vi "ATMEGA_Read_Write_labview.vi"() -> ()   [LabVIEW 2013]
doc: "This example performs writes and reads on a serial port, as directed by the user. You can press the Write and Read buttons, and change the Read Count, while the example is running.\n\nThe parameters set for the serial port must match the parameters of the connected instrument or device. In this example, the Read Count parameter specifies the number of bytes that the serial port reads. If there were more bytes at the port than the specified number, those bytes would not be read. If there were less bytes at the port than the specified number, you would receive a timeout error.\n\nThis example expands upon the flow control options for XON and XOFF, allowing the user to choose those control characters. Also, the user can enable or disable a termination character. Some devices require a termination character in order to identify the end of command strings. Some devices send a termination character to signify the end of data to be read. This example shows how you can end the Read operation once a termination character is detected in the buffer and/or append a termination character at the end of the Write data."
uses:
  D:/Program Files (x86)/National Instruments/LabVIEW 2013/examples/Instrument IO/Serial/support/Serial - Settings.ctl
  <vilib>/Instr/_visa.llb/VISA Configure Serial Port (Instr).vi
panel:
  out "Thermometer":dbl(slide) scale=0.0..500.0
  out "TEMP":i32
  out "READ BUFFER":string
  in  "write buffer":string
  in  "Stop":bool
  in  "Read Count":u32=1000
  out "Response":string
  in  "Write":bool
  in  "Read":bool
  in  "Serial Settings":T1={"baud rate"=9600, "data bits"=8, "parity"=enum."None", "stop bits"=10, "flow control"=0} {"flow control" items=["None"=0, "XON/XOFF"=1, "RTS/CTS"=2, "DTR/DSR"=4]; "stop bits" items=["1.0"=10, "1.5"=15, "2.0"=20]; "data bits" min=5 max=8 step=1; "baud rate" items=["75"=75, "110"=110, "134"=134, "150"=150, "300"=300, "600"=600, "1200"=1200, "1800"=1800, "2400"=2400, "4800"=4800, "7200"=7200, "9600"=9600, "14400"=14400, "19200"=19200, "28800"=28800, "38400"=38400, "56000"=56000, "57600"=57600, "115200"=115200, "128000"=128000, "230400"=230400]}
  in  "VISA resource name":refnum<visa-resource-name>="COM1"
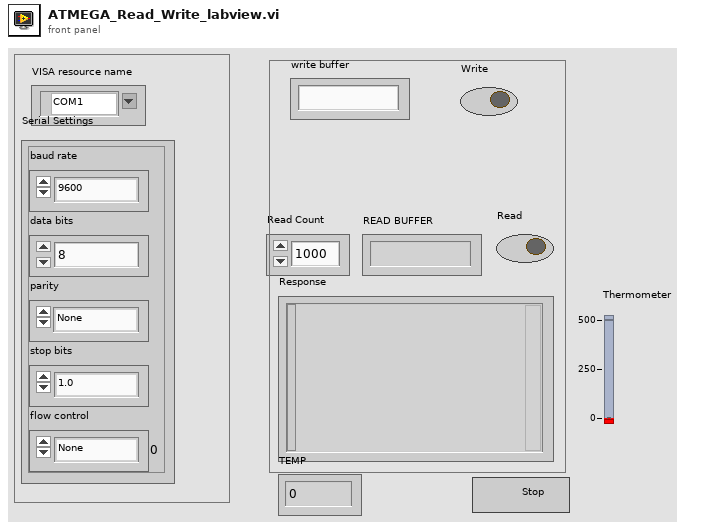
[diagram p1: front panel]
types:
  T1 = typedef "Serial - Settings.ctl" = cluster{"baud rate":u32, "data bits":u16, "parity":enum16{"None", "Odd", "Even", "Mark", "Space"}, "stop bits":u16, "flow control":u16}
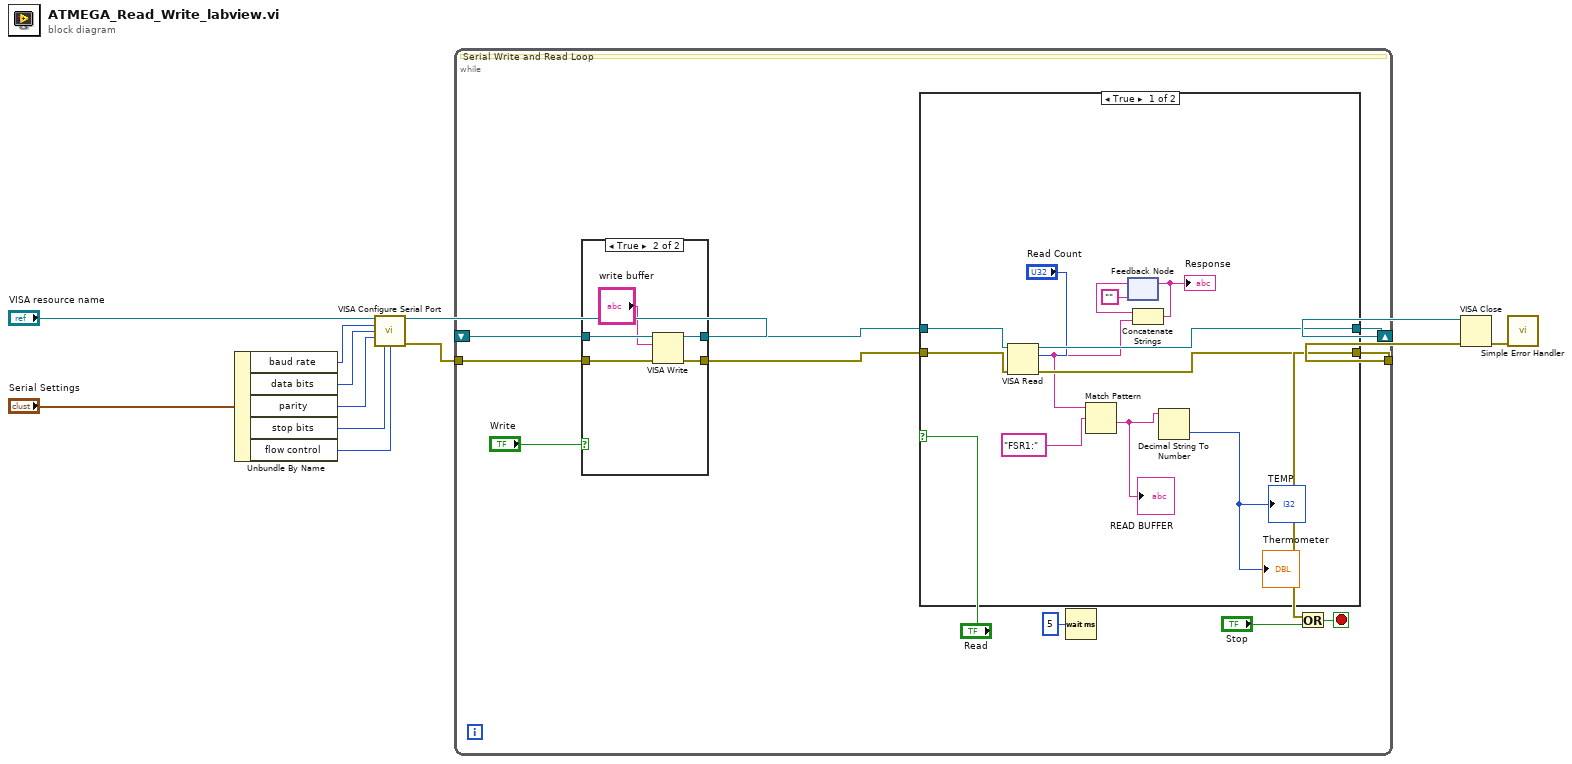
[diagram p0: block diagram]
diagram:
  n1 = Unbundle By Name "Unbundle By Name"("Serial Settings") -> ("baud rate"=w8:u32, "data bits"=w9:u16, "parity"=w10:enum16{"None", "Odd", "Even", "Mark", "Space"}, "stop bits"=w11:u16, "flow control"=w3:u16)
  n2 = call-poly "VISA Configure Serial Port"("VISA resource name"="VISA resource name", "baud rate (9600)"=w8, "data bits (8)"=w9, "parity (0:none)"=w10, "stop bits (10: 1 bit)"=w11, "flow control (0:none)"=w3) -> ("VISA resource name out"=w2:refnum<visa-resource-name>, "error out"=w1:errorcluster)  [unwired: 4 in, 4 out]
  n3 = while {
    shift-right: [w23] -> w4
    shift-left: w2 -> [w22]
    tunnel: [w16] -> w5
    tunnel: w1 -> [w13]
    stop <- w17 stop-if-true
    # "Serial Write and Read Loop"
    n4 = case shown="True" "Write" {
      tunnel: w22 -> [w25 w30]
      tunnel: w13 -> [w24 w29]
      tunnel: [w25 w28] -> w21
      tunnel: [w24 w27] -> w20
      frame False {
      }
      frame True {
        n5 = VISA Write(VISA resource name=w30, write buffer="write buffer", error in (no error)=w29) -> (VISA resource name out=w28:refnum<visa-resource-name>, error out=w27:errorcluster)  [unwired: 1 out]
      }
    }
    n6 = case shown="True" "Read" {
      tunnel: [w40 w44] -> w23
      tunnel: w21 -> [w42 w44]
      tunnel: [w38 w43] -> w16
      tunnel: w20 -> [w41 w43]
      frame True {
        n7 = VISA Read(VISA resource name=w42, byte count="Read Count", error in (no error)=w41) -> (VISA resource name out=w40:refnum<visa-resource-name>, read buffer=w34:string, error out=w38:errorcluster)  [unwired: 1 out]
        n8 = Match Pattern(string=w34, regular expression="FSR1:") -> (after substring=w32:string)  [unwired: 1 in, 3 out]
        "READ BUFFER" <- w32
        n9 = feedback #1("") -> (w37:string)
        n10 = Concatenate Strings(w37, w34) -> (w36:string)
        "Response" <- w36
        n11 = feedback-in #1(w36) -> ()
        n12 = Decimal String To Number(string=w32) -> (number=→"TEMP" →"Thermometer":i32)  [unwired: 2 in, 1 out]
      }
      frame False {
      }
    }
    n13 = Wait (ms)(milliseconds to wait=u32 5) -> ()  [unwired: 1 out]
    n14 = Or(x=w16, y="Stop") -> (x .or. y?=w17:bool)
  }
  n15 = VISA Close(VISA resource name=w4, error in (no error)=w5) -> (error out=w6:errorcluster)
  n16 = call <vilib>:"Simple Error Handler.vi"("error in (no error)"=w6) -> ()  [unwired: 1 in, 8 out]
